vi "TXTX niScope Measure Phase Stability.vi"() -> ()   [LabVIEW 2019]
doc: "Recommended Input Signal: 100 kHz, 4 Vpp, sine wave\n\nDevices Supported: Refer to NI Example Finder\n\nThis example configures all the oscilloscope's vertical, horizontal, and triggering properties before every acquisition. It allows you to experiment with numerous configurations, including acquisition types and triggering modes, since it supports nearly the entire functionality of NI-SCOPE. However, it is may be more instructive to consult other examples about specific topics such as FlexRes, Random Interleaved Sampling, and Multi-Record to learn more about these features.\n\nMany parameters are included an the front panel of this example. Notice that the \"min sample rate\" is next to the \"actual sample rate,\" and similarly the \"min record length\" is near the \"actual record length.\" The \"min\" values are specified with the Configure Horizontal Timing VI. NI-SCOPE maintains a constant time per record for each acquisition. So when you specify a min sample rate and a min record length, this determines the amount of time the acquisition should take:\n\n time per record = min record length / min sampling rate. \n\nHowever, oscilloscopes support only a certain number of defined sampling rates, so if the value chosen is not a valid rate, it is rounded to the next higher rate, called the actual sample rate. The actual record length is then calculated in order to maintain the time per record. Both of these values are returned in this example so you can investigate the effects of parameter rounding with your oscilloscope. For more information about parameter coercions, see the NI High Speed Digitizers Help.\n\nThe enforce realtime property allows this example to use Random Interleaved Sampling. See the Random Interleaved Sampling example for more details.\n\nKeep in mind that not all digitizers/oscilloscopes support all the features in this example. The NI High Speed Digitizers Help includes a table of supported features for each device."
uses:
  <vilib>/Analysis/NI_AALBase.lvlib
  <vilib>/measure/NI_MAPro.lvlib
  <vilib>/Analysis/NI_AALPro.lvlib
  <vilib>/Analysis/1siggen.llb/Ramp Pattern by Delta.vi
  <instrlib>/niScope/Configure/Trigger/niScope Configure Trigger Window.vi
  <instrlib>/niScope/Acquire/Fetch/niScope Multi Fetch WDT.vi
  <instrlib>/niScope/Configure/Trigger/niScope Configure Trigger Hysteresis.vi
  <vilib>/measure/matone.llb/Extract Single Tone Information N Chan.vi
  <instrlib>/niScope/Configure/Trigger/niScope Configure Trigger Digital.vi
  <instrlib>/niScope/Utility/niScope Get Channel Name From String.vi
  <vilib>/Utility/file.llb/Write Delimited Spreadsheet (DBL).vi
  <instrlib>/niScope/Configure/Trigger/niScope Configure Trigger Edge.vi
  <instrlib>/niScope/Configure/Trigger/niScope Configure Trigger Immediate.vi
panel:
  out "Current Frequency Under Test":dbl=1000000000.0 format="%#_6p"
  out "Results":T1(array[cluster])=[{"frequency (Hz)"=10000000.0, "mean skew"=2.0836910231183513e-10, "skew std dev"=2.5614322059634387e-11, "skew pk-pk"=7.432518925075383e-11, "skews"=[1.739664629612937e-10, 1.8550404541600728e-10, 1.9018541658980194e-10, 2.2842244695799065e-10, 2.404837484685102e-10, 2.482916522120475e-10, 2.0548471666715317e-10, 2.2268316489875913e-10, 1.8353182264462166e-10, 2.0513754630216602e-10]}, {"frequency (Hz)"=50000000.0, "mean skew"=-2.5452516580558666e-11, "skew std dev"=3.4978058538239445e-12, "skew pk-pk"=1.1209334964554319e-11, "skews"=[-2.3349803310721994e-11, -2.6572696199206285e-11, -2.2208073327012193e-11, -2.766990723352172e-11, -2.3423157412656305e-11, -2.872578105645893e-11, -3.1108023305200086e-11, -1.9898688340645768e-11, -2.8141380161559348e-11, -2.3427655458604015e-11]}, {"frequency (Hz)"=100000000.0, "mean skew"=4.250346384836178e-11, "skew std dev"=1.5968033389031761e-12, "skew pk-pk"=4.752448395132127e-12, "skews"=[4.320489816934278e-11, 4.1510150659626536e-11, 4.246669542854741e-11, 4.1510386784212196e-11, 4.008805895264478e-11, 4.076342033154444e-11, 4.2166791318990814e-11, 4.4260094386458757e-11, 4.484050734777691e-11, 4.422363510447316e-11]}, {"frequency (Hz)"=150000000.0, "mean skew"=3.048616518608692e-11, "skew std dev"=2.0348946116357876e-12, "skew pk-pk"=5.743552157363673e-12, "skews"=[3.008035096882213e-11, 3.37166407550793e-11, 3.063833874904634e-11, 2.7973088597715625e-11, 3.0352657349370103e-11, 2.8615049954055002e-11, 3.215931135439043e-11, 2.8165315277876678e-11, 3.334513374168875e-11, 2.981576511282481e-11]}, {"frequency (Hz)"=200000000.0, "mean skew"=1.7233054218079923e-11, "skew std dev"=1.2623091696220342e-12, "skew pk-pk"=4.0297344588068415e-12, "skews"=[1.7728536107607546e-11, 1.5111641064571448e-11, 1.6505201591003324e-11, 1.7835612302818712e-11, 1.625886715101237e-11, 1.6287520534090016e-11, 1.8410179041316403e-11, 1.8436926097106544e-11, 1.914137552337829e-11, 1.661468276789457e-11]}, {"frequency (Hz)"=250000000.0, "mean skew"=2.6392233367607176e-11, "skew std dev"=8.681273640938131e-13, "skew pk-pk"=2.8373944155729497e-12, "skews"=[2.6700638621598095e-11, 2.5532836606242813e-11, 2.7334856846612955e-11, 2.5053029280374876e-11, 2.6617693547116632e-11, 2.6122214073676364e-11, 2.6834184000852343e-11, 2.62746862964246e-11, 2.7890423695947825e-11, 2.5561770707225246e-11]}, {"frequency (Hz)"=300000000.0, "mean skew"=3.5715499673422923e-11, "skew std dev"=9.22303373657949e-13, "skew pk-pk"=2.4396817696088776e-12, "skews"=[3.680447374590992e-11, 3.543915094779086e-11, 3.5048085347651886e-11, 3.4641319268602025e-11, 3.460188140866298e-11, 3.565680633749764e-11, 3.704156317827186e-11, 3.677877545548181e-11, 3.6128325034950285e-11, 3.501461600941e-11]}, {"frequency (Hz)"=350000000.0, "mean skew"=2.9742763156759984e-11, "skew std dev"=1.5760453786816616e-12, "skew pk-pk"=5.3732542947032374e-12, "skews"=[2.8992495989930434e-11, 2.935337910903846e-11, 2.862552296924053e-11, 3.060069745802097e-11, 2.954847865308417e-11, 2.8236706740636113e-11, 3.104203003443178e-11, 3.2873164424420016e-11, 3.065524605908058e-11, 2.749991012971678e-11]}, {"frequency (Hz)"=400000000.0, "mean skew"=2.6733516663180105e-11, "skew std dev"=1.10810830482662e-12, "skew pk-pk"=3.4502418977022077e-12, "skews"=[2.542949644854753e-11, 2.5980255035497056e-11, 2.7914995058437394e-11, 2.7345747276370938e-11, 2.599715484539292e-11, 2.6683690871151727e-11, 2.6740144484632127e-11, 2.8646662117202237e-11, 2.7400600275069104e-11, 2.519642021950003e-11]}, {"frequency (Hz)"=450000000.0, "mean skew"=3.1133628207442694e-11, "skew std dev"=9.848098089565015e-13, "skew pk-pk"=3.0907132712086158e-12, "skews"=[3.0516817875288693e-11, 3.116049803538605e-11, 3.113864358328799e-11, 3.253802361259391e-11, 3.2693079811960275e-11, 3.111382674392098e-11, 3.095760801909229e-11, 3.163070682932932e-11, 2.998471102281578e-11, 2.960236654075166e-11]}, {"frequency (Hz)"=500000000.0, "mean skew"=2.5573986101229784e-11, "skew std dev"=1.2520536533547348e-12, "skew pk-pk"=4.028404853675228e-12, "skews"=[2.623305513695395e-11, 2.3069415018043377e-11, 2.5710709926330432e-11, 2.695097571714925e-11, 2.7097819871718605e-11, 2.4318053879682445e-11, 2.579175772512857e-11, 2.5465682737947023e-11, 2.467738916537633e-11, 2.642500183396782e-11]}, {"frequency (Hz)"=550000000.0, "mean skew"=1.5567566299195614e-11, "skew std dev"=7.67007037754582e-13, "skew pk-pk"=2.454609815510684e-12, "skews"=[1.546343560548785e-11, 1.5691991339421908e-11, 1.4763651327091542e-11, 1.5656995661825636e-11, 1.4352486372154259e-11, 1.6807096187664943e-11, 1.4703999473694154e-11, 1.5863442067828158e-11, 1.615212584270498e-11, 1.6220439114082706e-11]}, {"frequency (Hz)"=600000000.0, "mean skew"=1.0960985352102524e-11, "skew std dev"=1.5158264044949614e-12, "skew pk-pk"=4.417736521406017e-12, "skews"=[1.034865241465638e-11, 9.15607462098645e-12, 1.3080874575270249e-11, 1.1362167251477812e-11, 9.435856668762349e-12, 1.072321135118218e-11, 1.3573811142392468e-11, 1.1065725009931054e-11, 9.289056595931725e-12, 1.1574423890434564e-11]}, {"frequency (Hz)"=650000000.0, "mean skew"=1.1785798816628399e-11, "skew std dev"=1.8374886424553172e-12, "skew pk-pk"=5.803228144519101e-12, "skews"=[1.3765488156165523e-11, 1.527024540782444e-11, 1.1115487041155591e-11, 1.0788052994466733e-11, 1.2159650690597356e-11, 1.2811035279136584e-11, 9.467017263305338e-12, 9.656035886946132e-12, 1.0546551042843003e-11, 1.2278424403843278e-11]}, {"frequency (Hz)"=700000000.0, "mean skew"=6.596076318740604e-12, "skew std dev"=8.641094493766275e-13, "skew pk-pk"=2.9349975398458985e-12, "skews"=[6.115659901924894e-12, 6.3426614341559345e-12, 6.8334690852228706e-12, 6.6351686442937046e-12, 8.012367711317768e-12, 6.338949209907351e-12, 5.785725677118076e-12, 7.47364327887804e-12, 5.0773701714718694e-12, 7.345748073115535e-12]}, {"frequency (Hz)"=750000000.0, "mean skew"=-8.004232000094917e-13, "skew std dev"=1.9589852308635695e-12, "skew pk-pk"=5.878410167209685e-12, "skews"=[-2.0043424970715243e-12, -2.060546126274997e-12, 1.7757154794342005e-12, -3.403103182827954e-12, -8.375922075224257e-13, -6.352730610550562e-13, -1.6564006068083883e-12, 9.872406366440281e-13, -2.6452374189945313e-12, 2.4753069843817308e-12]}, {"frequency (Hz)"=800000000.0, "mean skew"=-1.1908329622689498e-12, "skew std dev"=2.4471655381374184e-12, "skew pk-pk"=7.571440643406824e-12, "skews"=[-2.702444448534128e-12, -4.492699533766456e-12, -1.277443678925676e-12, 1.2013408188686924e-12, -5.465462251255593e-12, -8.479963637763869e-13, 4.460986499403048e-13, 2.1059783921512303e-12, 5.38831539272422e-13, -1.4145327466639087e-12]}, {"frequency (Hz)"=850000000.0, "mean skew"=3.205551700745509e-12, "skew std dev"=3.0129265707549263e-12, "skew pk-pk"=9.163933099015031e-12, "skews"=[-2.13224713394751e-13, 8.279216091294899e-13, 4.100539825167484e-12, 3.12742661061994e-12, 3.0112015228428608e-12, -5.305439632819706e-13, 3.2381630888442507e-12, 2.27109799246451e-12, 7.589545899330212e-12, 8.63338913573306e-12]}, {"frequency (Hz)"=900000000.0, "mean skew"=2.7489377497772397e-12, "skew std dev"=3.2558595326691925e-12, "skew pk-pk"=1.1255800529200094e-11, "skews"=[7.673148096180858e-12, -7.002449595507266e-13, 4.223614561545406e-12, 1.4310789419395444e-12, 4.3512183242227034e-12, -3.582652433019236e-12, 2.3464731912235006e-12, 6.248694181205894e-12, 2.3729592170649844e-12, 3.125088376959467e-12]}, {"frequency (Hz)"=950000000.0, "mean skew"=-4.302246450539571e-12, "skew std dev"=3.422107033759102e-12, "skew pk-pk"=1.1002162963748398e-11, "skews"=[-6.151157544668618e-12, -6.928006418031253e-12, -6.495629316988361e-13, -2.2617091792843392e-13, -5.581516495423095e-12, -4.445735673178396e-12, -4.7377111659940605e-12, -1.1228333881676832e-11, -1.4405700214015436e-12, -1.6336994553946392e-12]}, {"frequency (Hz)"=1000000000.0, "mean skew"=-1.680303661322012e-13, "skew std dev"=1.7303427813605274e-12, "skew pk-pk"=5.7763544962238485e-12, "skews"=[-1.221791759348109e-12, 1.4506889878445898e-12, -2.0644323940287416e-12, -3.148191138723442e-12, 1.6919563689652573e-15, 2.6281633575004064e-12, 1.6032209001872605e-13, 2.71957331308119e-13, 1.2212882479375565e-12, -9.800003402000824e-13]}] {"frequency (Hz)" format="%#_6p"; "mean skew" format="%#_6p"; "skew std dev" format="%#_6p"; "skew pk-pk" format="%#_6p"; "skews" format="%#_6p"}
  in  "iterations":i32=10
  in  "Trigger Type":T2(tab)
  in  "Trigger Source":string(combo)="0"
  in  "Trigger Level":dbl format="%.2f"
  in  "Trigger Slope":i32(ring) items=["Positive", "Negative"]
  in  "Coupling":u16(ring)=1 caption="Trigger Coupling" items=["AC"=0, "DC"=1, "HF Reject"=3, "LF Reject"=4, "AC Plus HF Reject"=1001]
  in  "Trigger Slope":i32(ring) items=["Positive", "Negative"]
  in  "Trigger Source":string(combo)="VAL_PFI_1"
  in  "Coupling":u16(ring)=1 caption="Trigger Coupling" items=["AC"=0, "DC"=1, "HF Reject"=3, "LF Reject"=4, "AC Plus HF Reject"=1001]
  in  "High Level":dbl=0.1 caption="Window High Level" format="%.2f"
  in  "Low Level":dbl=-0.1 caption="Window Low Level" format="%.2f"
  in  "Window Mode":i32(ring) items=["Entering", "Leaving"]
  in  "Trigger Source":string(combo)="0"
  in  "Hysteresis":dbl=0.05 format="%.2f"
  in  "Trigger Source":string(combo)="0"
  in  "Trigger Level":dbl format="%.2f"
  in  "Coupling":u16(ring)=1 caption="Trigger Coupling" items=["AC"=0, "DC"=1, "HF Reject"=3, "LF Reject"=4, "AC Plus HF Reject"=1001]
  in  "Trigger Slope":i32(ring) items=["Positive", "Negative"]
  out "Auto Triggered":bool
  in  "Trigger Modifier":i32(ring)=2 items=["None"=1, "Auto Trigger"=2]
  in  "Vertical Coupling":i32(ring)=1 items=["AC", "DC", "Ground"]
  in  "Stop":bool
  in  "Reference Position":dbl=50.0 caption="Ref Position" format="%.1f"
  in  "Trigger Delay":dbl caption="Trigger Delay (s)" format="%#.4p"
  in  "Maximum Input Frequency":dbl=-1.0 caption="Max. Input Frequency (Hz)" format="%.2p"
  in  "Input Impedance":u32(ring) items=["1 mega ohm"=0, "50 ohms"=2]
  in  "Probe Attenuation":dbl=1.0 format="%.1f"
  in  "Vertical Offset":dbl caption="Vertical Offset (V)" format="%.2p"
  in  "Timeout (s)":dbl=5.0 caption="Timeout(s)" format="%.2f"
  out "Actual Sample Rate":dbl=2500000000.0 format="%#.2p"
  out "Actual Record Length":i32=1000
  out "Waveform(s)":waveform(dbl)[](graph)
  in  "Min Record Length":i32=1000 caption="Min. Record Length"
  in  "Min Sample Rate":dbl=2500000000.0 caption="Min. Sample Rate" step=1000000.0 format="%#.2p"
  in  "Vertical Range":dbl=1.0 caption="Vertical Range (V)" format="%.2f"
  in  "Enforce Realtime":bool=TRUE
  in  "Channel Name":string="0,1" caption="Channel(s)"
  in  "Resource Name":refnum<k15>="PXI1Slot3" caption="Resource Name(s)"
  # "Vertical"
  # "Channel"
  # "Trigger"
  # "Common Trigger Settings"
  # "Horizontal"
  # "Note: When configured for Immediate reference trigger, this example does not configure any additional trigger settings - the acquisition is triggered as soon as possible after being initiated by driver software."
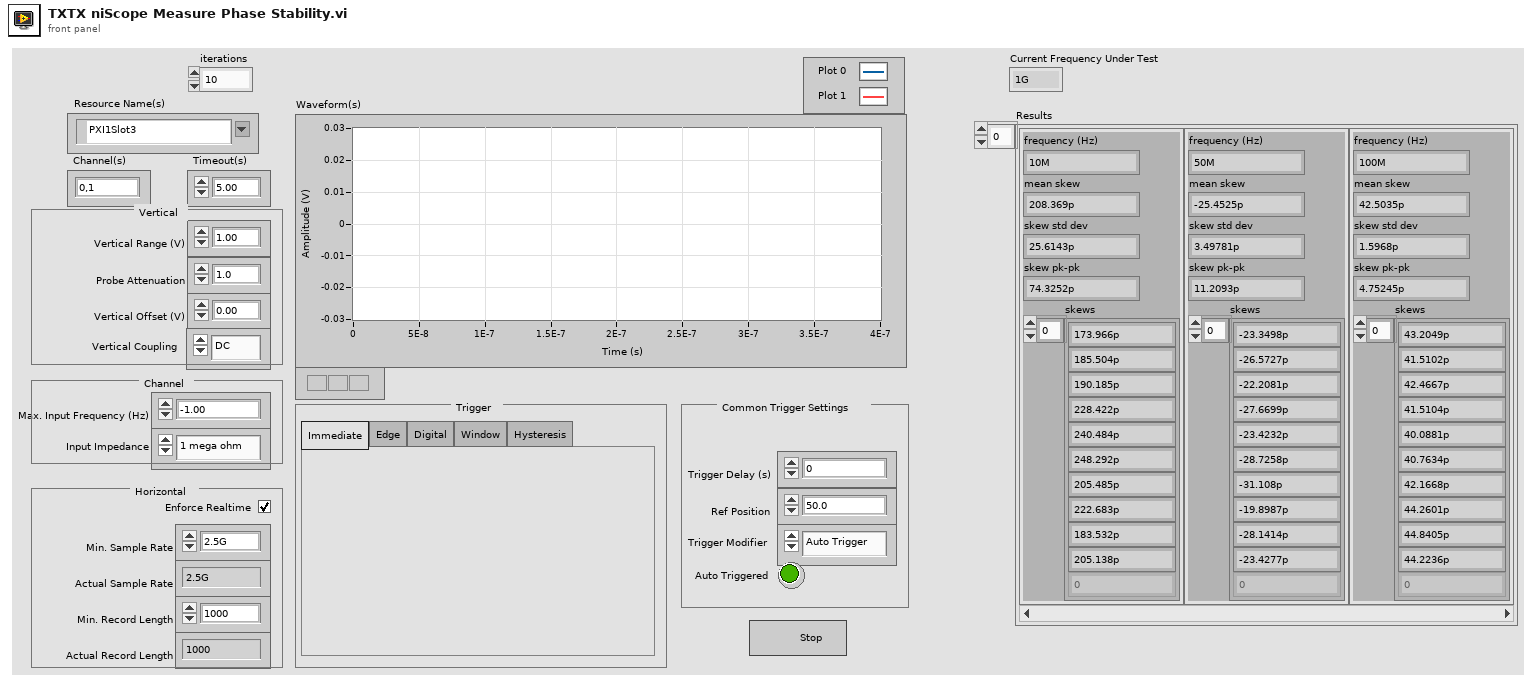
[diagram p1: front panel]
types:
  T1 = cluster{"frequency (Hz)":dbl, "mean skew":dbl, "skew std dev":dbl, "skew pk-pk":dbl, "skews":dbl[]}[]
  T2 = enum32{"Immediate", "Edge", "Digital", "Window", "Hysteresis"}
  T3 = cluster{"frequency":dbl, "mean skew":dbl, "skew std dev":dbl, "skew pk-pk":dbl, "skews":dbl[]}
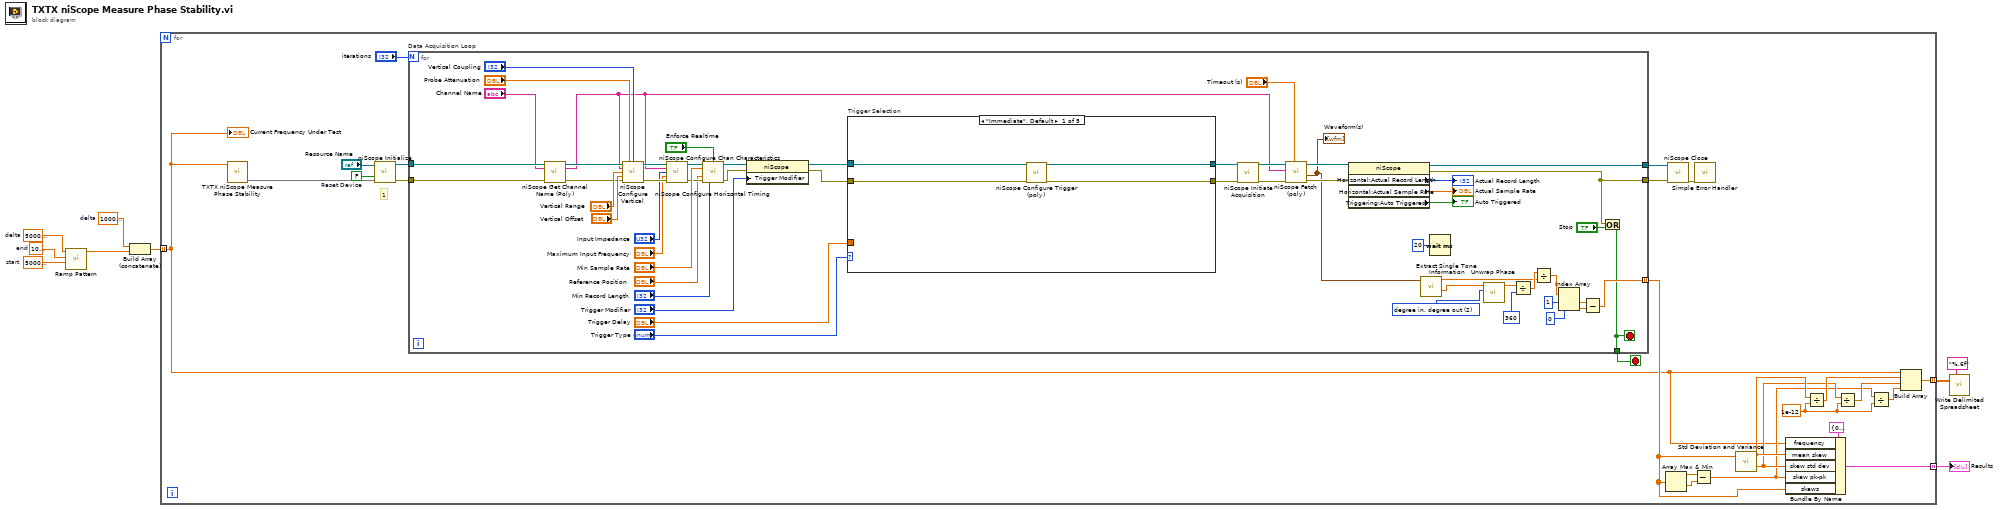
[diagram p0: block diagram]
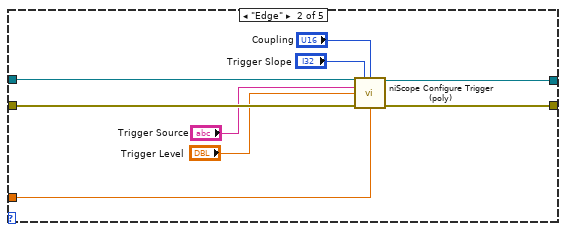
[diagram p2: hidden frame]
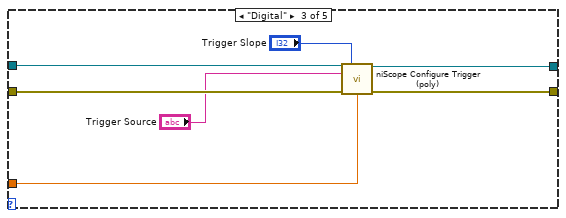
[diagram p3: hidden frame]
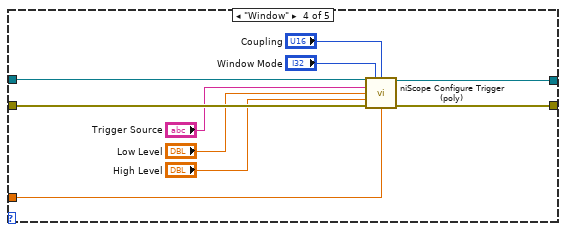
[diagram p4: hidden frame]
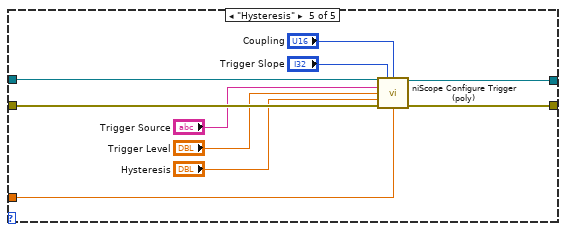
[diagram p5: hidden frame]
diagram:
  w2 = 10000000.0  # delta
  w7 = 50000000.0  # delta
  w8 = 1000000000.0  # end
  w9 = 50000000.0  # start
  n1 = call-poly <vilib>:"Ramp Pattern.vi"("start"=w9, "end"=w8, "delta"=w7) -> ("Ramp Pattern"=w4:dbl[])  [unwired: 6 in, 2 out]
  n2 = Build Array (concatenate)(w2, w4) -> (w3:dbl[])
  n3 = for {
    tunnel: [w24] -> w5 mode=indexing
    tunnel: [w23] -> w6 mode=indexing
    tunnel: w3 -> [w10] mode=indexing
    stop <- w21 stop-if-true
    w11 = 1e-12 ("y")
    w33 = FALSE  # Reset Device
    # "1"
    n4 = call "TXTX niScope Measure Phase Stability.vi"(11:w10) -> (0:w22)  [unwired: 10 in]
    n5 = call <instrlib>:"niScope Initialize.vi"("resource name"="Resource Name", "reset device"=w33, "error in"=w22) -> ("instrument handle"=w30:refnum<k15>, "error out"=w27:errorcluster)  [unwired: 11 in]
    n6 = for "Data Acquisition Loop" {
      N: "iterations" -> [_]
      tunnel: [w60] -> w31
      tunnel: w30 -> [w53]
      tunnel: w27 -> [w50]
      tunnel: [w54] -> w29
      tunnel: [w42] -> w25 mode=indexing
      tunnel: [w37] -> w21
      stop <- w37 stop-if-true
      w40 = 2 items=["radian in, radian out", "radian in, degree out", "degree in, degree out", "degree in, radian out"] ("phase unit")
      n7 = call-poly <instrlib>:"niScope Get Channel Name (Poly).vi"("instrument handle"=w53, "index"="Channel Name", "error in"=w50) -> ("instrument handle out"=w52:refnum<k15>, "channel name"=w48:string, "error out"=w51:errorcluster)  [unwired: 10 in]
      n8 = call <instrlib>:"niScope Configure Vertical.vi"("instrument handle"=w52, "probe attenuation"="Probe Attenuation", "vertical coupling"="Vertical Coupling", "channels"=w48, "vertical range"="Vertical Range", "vertical offset"="Vertical Offset", "error in"=w51) -> ("instrument handle out"=w85:refnum<k15>, "error out"=w84:errorcluster)  [unwired: 7 in]
      n9 = call <instrlib>:"niScope Configure Chan Characteristics.vi"("instrument handle"=w85, "channels"=w48, "input impedance"="Input Impedance", "maximum input frequency"="Maximum Input Frequency", "error in"=w84) -> ("instrument handle out"=w82:refnum<k15>, "error out"=w83:errorcluster)  [unwired: 9 in]
      n10 = call <instrlib>:"niScope Configure Horizontal Timing.vi"("instrument handle"=w82, "enforce realtime"="Enforce Realtime", "min sample rate"="Min Sample Rate", "reference position"="Reference Position", "error in"=w83, "min record length"="Min Record Length") -> ("instrument handle out"=w67:refnum<k15>, "error out"=w66:errorcluster)  [unwired: 8 in]
      n11 = property on="Property Node" class="niScope"(reference=w67, error in=w66, "Trigger Modifier"="Trigger Modifier") -> (reference out=w64:refnum<k15>, error out=w65:errorcluster)
      n12 = case "Trigger Selection" shown="\"Immediate\", Default" "Trigger Type" {
        tunnel: w65 -> [w92 w101 w108 w118 w128]
        tunnel: [w89 w97 w104 w114 w124] -> w70
        tunnel: w64 -> [w91 w100 w107 w117 w127]
        tunnel: [w90 w98 w105 w115 w126] -> w73
        tunnel: "Trigger Delay" -> [_ w99 w106 w116 w125]
        frame "Immediate", Default {
          n13 = call-poly <instrlib>:"niScope Configure Trigger (poly).vi"("instrument handle"=w91, "error in"=w92) -> ("instrument handle out"=w90:refnum<k15>, "error out"=w89:errorcluster)  [unwired: 12 in]
        }
        frame "Edge" {
          n14 = call-poly <instrlib>:"niScope Configure Trigger (poly).vi"("instrument handle"=w100, "trigger slope"="Trigger Slope", "trigger coupling"="Coupling", "trigger source"="Trigger Source", "trigger level"="Trigger Level", "error in"=w101, "trigger delay"=w99) -> ("instrument handle out"=w98:refnum<k15>, "error out"=w97:errorcluster)  [unwired: 7 in]
        }
        frame "Digital" {
          n15 = call-poly <instrlib>:"niScope Configure Trigger (poly).vi"("instrument handle"=w107, "trigger slope"="Trigger Slope", "trigger source"="Trigger Source", "error in"=w108, "trigger delay"=w106) -> ("instrument handle out"=w105:refnum<k15>, "error out"=w104:errorcluster)  [unwired: 9 in]
        }
        frame "Window" {
          n16 = call-poly <instrlib>:"niScope Configure Trigger (poly).vi"("instrument handle"=w117, "trigger window mode"="Window Mode", "trigger coupling"="Coupling", "trigger source"="Trigger Source", "low level"="Low Level", "high level"="High Level", "error in"=w118, "trigger delay"=w116) -> ("instrument handle out"=w115:refnum<k15>, "error out"=w114:errorcluster)  [unwired: 6 in]
        }
        frame "Hysteresis" {
          n17 = call-poly <instrlib>:"niScope Configure Trigger (poly).vi"("instrument handle"=w127, "trigger slope"="Trigger Slope", "trigger coupling"="Coupling", "trigger source"="Trigger Source", "trigger level"="Trigger Level", "hysteresis"="Hysteresis", "error in"=w128, "trigger delay"=w125) -> ("instrument handle out"=w126:refnum<k15>, "error out"=w124:errorcluster)  [unwired: 6 in]
        }
      }
      n18 = call <instrlib>:"niScope Initiate Acquisition.vi"("instrument handle"=w73, "error in"=w70) -> ("instrument handle out"=w72:refnum<k15>, "error out"=w71:errorcluster)  [unwired: 12 in]
      n19 = call-poly <instrlib>:"niScope Fetch (poly).vi"("timeout"="Timeout (s)", "error in"=w71, "channels"=w48, "instrument handle"=w72) -> ("error out"=w61:errorcluster, "wfm"=w41:waveform(dbl)[], "instrument handle out"=w62:refnum<k15>)  [unwired: 4 in, 1 out]
      "Waveform(s)" <- w41
      n20 = property class="niScope"(reference=w62, error in=w61) -> (reference out=w60:refnum<k15>, error out=w54:errorcluster, "Horizontal:Actual Record Length"=→"Actual Record Length":i32, "Horizontal:Actual Sample Rate"=→"Actual Sample Rate":dbl, "Triggering:Auto Triggered"=→"Auto Triggered":bool)
      n21 = call-poly <vilib>:"Extract Single Tone Information.vi"("time signals in"=w41) -> ("detected phases (deg)"=w39:dbl[], "detected frequencies"=w43:dbl[])  [unwired: 5 in, 4 out]
      n22 = Wait (ms)(milliseconds to wait=u32 20) -> ()  [unwired: 1 out]
      n23 = call <vilib>:"Unwrap Phase.vi"("phase unit"=w40, "Phase"=w39) -> ("Unwrapped Phase"=w47:dbl[])  [unwired: 8 in, 1 out]
      n24 = Divide(x=w47, y=360) -> (x/y=w46:dbl[])
      n25 = Divide(x=w46, y=w43) -> (x/y=w44:dbl[])
      n26 = Index Array(array=w44, index #1=1 ("index (row)"), index #2=0 ("index (row)")) -> (element #1=w35:dbl, element #2=w34:dbl)
      n27 = Subtract(x=w35, y=w34) -> (x-y=w42:dbl)
      n28 = Or(x=w54, y="Stop") -> (x .or. y?=w37:bool)
    }
    n29 = Array Max & Min(array=w25) -> (max value=w19:dbl, min value=w20:dbl)  [unwired: 2 out]
    n30 = call <instrlib>:"niScope Close.vi"("instrument handle"=w31, "error in"=w29) -> ("error out"=w32:errorcluster)  [unwired: 13 in]
    n31 = Subtract(x=w19, y=w20) -> (x-y=w13:dbl)
    n32 = call <vilib>:"Simple Error Handler.vi"("error in (no error)"=w32) -> ()  [unwired: 4 in, 5 out]
    n33 = call <vilib>:"Std Deviation and Variance.vi"("X"=w25) -> ("mean"=w17:dbl, "standard deviation"=w15:dbl)  [unwired: 1 in, 1 out]
    n34 = Bundle By Name(cluster=T3 {"frequency"=0.0, "mean skew"=0.0, "skew std dev"=0.0, "skew pk-pk"=0.0, "skews"=[]}, "frequency"=w10, "mean skew"=w17, "skew std dev"=w15, "skew pk-pk"=w13, "skews"=w25) -> (w23:T3)
    n35 = Divide(x=w17, y=w11) -> (x/y=w16:dbl)
    n36 = Divide(x=w15, y=w11) -> (x/y=w14:dbl)
    n37 = Divide(x=w13, y=w11) -> (x/y=w12:dbl)
    n38 = Build Array(w10, w16, w14, w12) -> (w24:dbl[])
    "Current Frequency Under Test" <- w10
  }
  "Results" <- w6
  n39 = call-poly <vilib>:"Write Delimited Spreadsheet.vi"("format (%.3f)"="%.6f", "2D data"=w5) -> ()  [unwired: 12 in, 2 out]
